vi "setHQtime.vi"   [LabVIEW 2014]
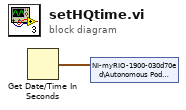
[diagram p0: block diagram]
diagram:
  n1 = Get Date/Time In Seconds() -> (seconds since 1Jan1904=w1:timestamp)
  n2 = shared-variable "NI-myRIO-1900-030d70ed\\Autonomous Pod Shared Variables.lvlib\\HqTime"(w1) -> ()  [unwired: 1 in, 1 out]
